vi "AccountsFileAccess (SubVI).vi"(7 "AccountCommand":T1, 8 "Error In":errorcluster, 10 "Parcel number":string, 11 "Phone number":string) -> (0 "Error Out":errorcluster, 1 "Parcel locker":string, 2 "Phone number":string, 3 "Parcel number":string)   [LabVIEW 2017]
doc: "This VI manages the connection to the accounts file. Allows to find an account, make a deposit or withdrawal."
uses:
  Controls/AccountsFileCommand.ctl
  <vilib>/Utility/file.llb/Read From Spreadsheet File (string).vi
  GlobalPhoneNumber.vi
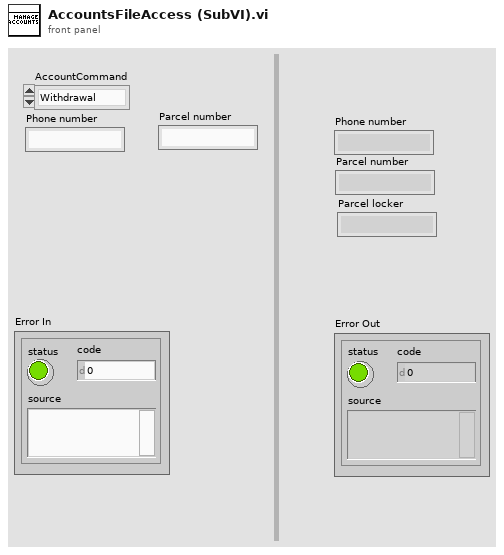
[diagram p1: front panel]
types:
  T1 = typedef "AccountsFileCommand.ctl" = enum16{"Withdrawal", "GetPhoneNumber", "Deposit", "GetParcelNumber"}
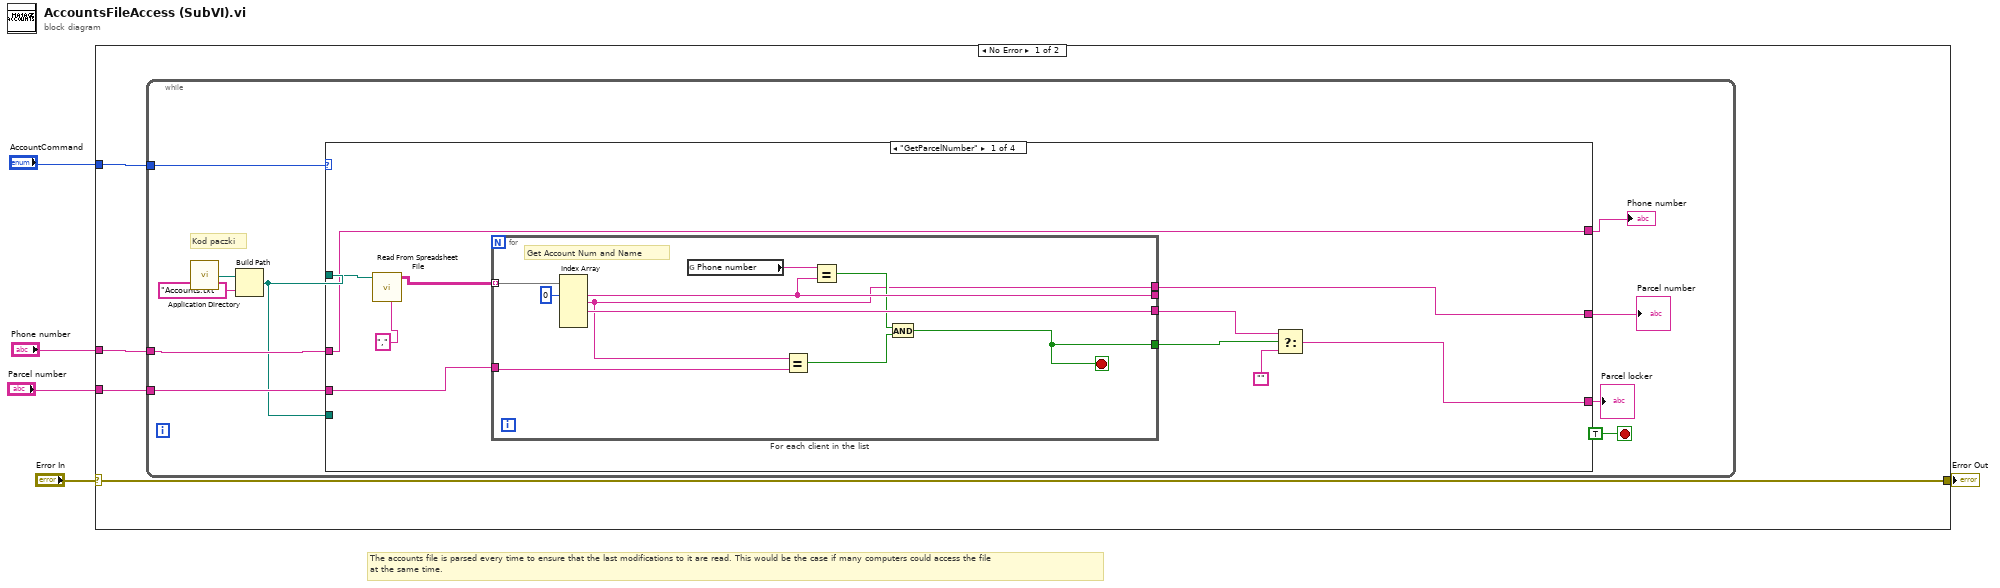
[diagram p0: block diagram]
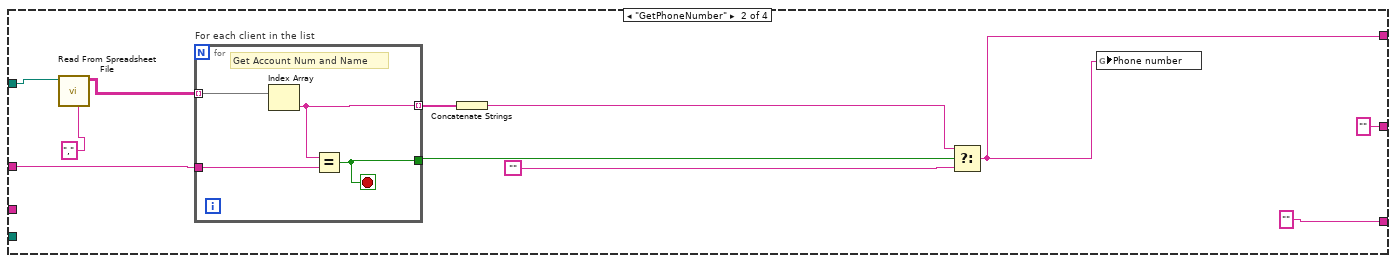
[diagram p2: hidden frame]
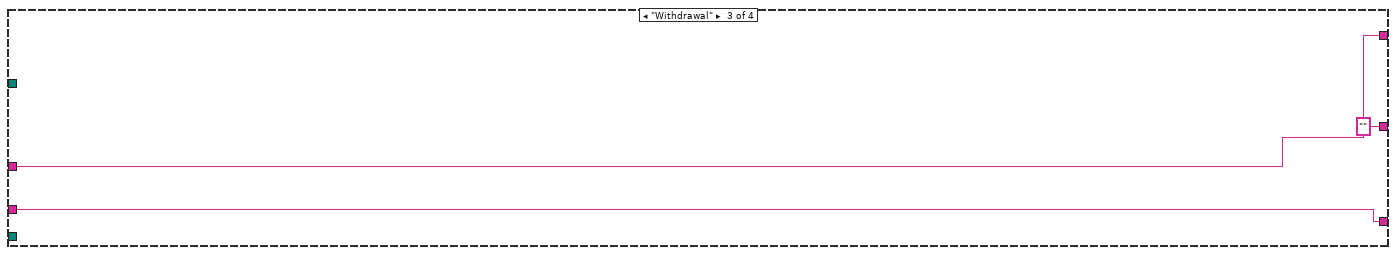
[diagram p3: hidden frame]
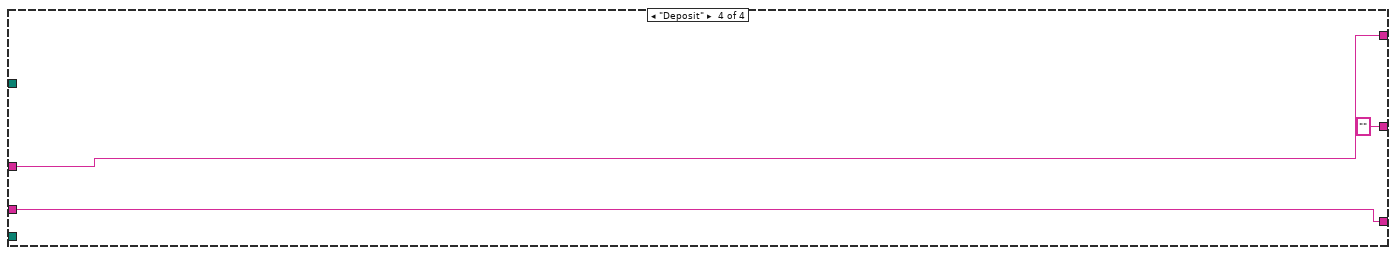
[diagram p4: hidden frame]
diagram:
  # "The accounts file is parsed every time to ensure that the last modifications to it are read. This would be the case if many computers could access the file\nat the same time."
  n1 = case shown="No Error" "Error In" {
    selector: "Error In" -> [w8 w61]
    tunnel: [w8 w61] -> w4
    tunnel: "Phone number" -> [w9 _]
    tunnel: "AccountCommand" -> [w7 _]
    tunnel: "Parcel number" -> [w6 _]
    frame No Error {
      n2 = while {
        tunnel: w9 -> [w14]
        tunnel: w7 -> [w16]
        tunnel: w6 -> [w15]
        stop <- TRUE stop-if-true
        # "Kod paczki"
        n3 = call <vilib>:"Application Directory.vi"() -> ("Application Directory"=w18:path)
        n4 = Build Path(base path=w18, name or relative path="Accounts.txt") -> (appended path=w13:path)
        n5 = case shown="\"GetParcelNumber\"" w16 {
          tunnel: w15 -> [w29 _ w56 w59]
          tunnel: w13 -> [_ _ _ _]
          tunnel: w14 -> [w22 w47 w57 w60]
          tunnel: w13 -> [w26 w45 _ _]
          tunnel: [w22 w40 w57 w60] -> w12
          tunnel: [w23 "" ("Parcel number") w56 w59] -> w10
          tunnel: [w21 "" ("String") "" ("String") "" ("String")] -> w11
          frame "GetParcelNumber" {
            n6 = call-poly <vilib>:"Read From Spreadsheet File.vi"("delimiter (\\t)"="," ("delimiter (\\t)"), "file path (dialog if empty)"=w26) -> ("all rows"=w24:string[][])  [unwired: 5 in, 4 out]
            n7 = for "For each client in the list" {
              tunnel: w29 -> [w39]
              tunnel: [w31] -> w28
              tunnel: [w34] -> _
              tunnel: [w37] -> w20
              tunnel: w24 -> [w38] mode=indexing
              tunnel: [w30] -> w21
              stop <- w31 stop-if-true
              # "Get Account Num and Name"
              n8 = Index Array(array=w38, index #1=0 ("index")) -> (element #1=w34:string, element #2=w30:string, element #3=w37:string)  [unwired: 4 in, 2 out]
              n9 = global read "GlobalPhoneNumber.vi" "Phone number"() -> (w35:string)
              n10 = Equal?(x=w30, y=w39) -> (x = y?=w32:bool)
              n11 = Equal?(x=w35, y=w34) -> (x = y?=w33:bool)
              n12 = And(x=w33, y=w32) -> (x .and. y?=w31:bool)
            }
            n13 = Select(t=w20, s=w28, f="") -> (s? t:f=w23:string)
          }
          frame "GetPhoneNumber" {
            n14 = call-poly <vilib>:"Read From Spreadsheet File.vi"("delimiter (\\t)"="," ("delimiter (\\t)"), "file path (dialog if empty)"=w45) -> ("all rows"=w44:string[][])  [unwired: 5 in, 4 out]
            n15 = for "For each client in the list" {
              tunnel: w47 -> [w54]
              tunnel: [w53] -> w49
              tunnel: w44 -> [w52] mode=indexing
              tunnel: [w51] -> w48 mode=indexing
              stop <- w53 stop-if-true
              # "Get Account Num and Name"
              n16 = Index Array(array=w52) -> (element=w51:string)  [unwired: 1 in]
              n17 = Equal?(x=w51, y=w54) -> (x = y?=w53:bool)
            }
            n18 = Concatenate Strings(w48) -> (w43:string)
            n19 = Select(t=w43, s=w49, f="") -> (s? t:f=w40:string)
            n20 = global write "GlobalPhoneNumber.vi" "Phone number"(w40) -> ()
          }
          frame "Withdrawal" {
          }
          frame "Deposit" {
          }
        }
        "Phone number" <- w12
        "Parcel number" <- w11
        "Parcel locker" <- w10
      }
    }
    frame Error {
    }
  }
  "Error Out" <- w4
